vi "Report_backup.vi"(6 "Func ctl":enum16{"Backup Report", "Recover Report"}(ring), 8 "error in":errorcluster, 11 "DUT?":string="DUT1") -> (0 "error out":errorcluster)   [LabVIEW 2012]
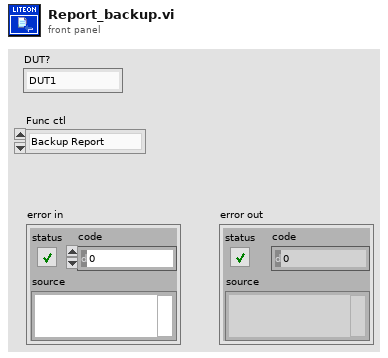
[diagram p1: front panel]
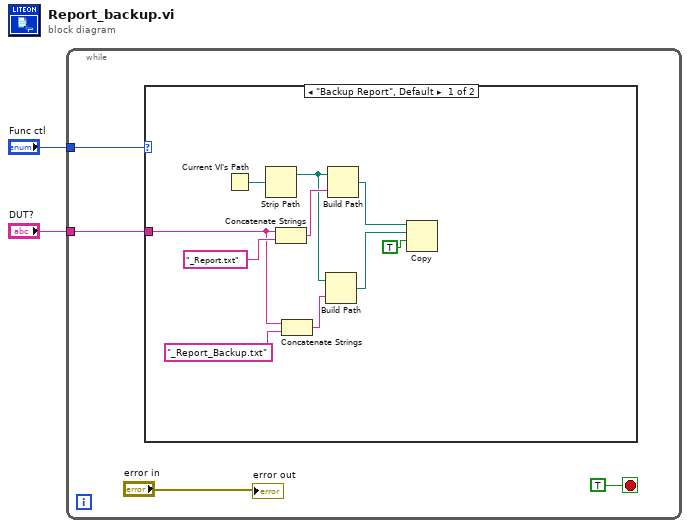
[diagram p0: block diagram]
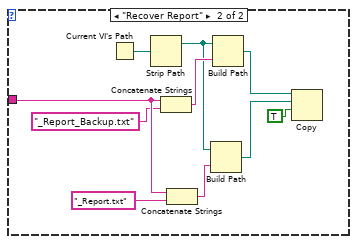
[diagram p2: hidden frame]
diagram:
  n1 = while {
    tunnel: "Func ctl" -> [w5]
    tunnel: "DUT?" -> [w4]
    stop <- TRUE stop-if-true
    n2 = case shown="\"Backup Report\", Default" w5 {
      tunnel: w4 -> [w7 w19]
      frame "Backup Report", Default {
        n3 = Current VI's Path() -> (path=w16:path)
        n4 = Strip Path(path=w16) -> (stripped path=w12:path)  [unwired: 1 out]
        n5 = Concatenate Strings(w7, "_Report.txt" ("string")) -> (w13:string)
        n6 = Concatenate Strings(w7, "_Report_Backup.txt" ("string")) -> (w11:string)
        n7 = Build Path(base path=w12, name or relative path=w11) -> (appended path=w9:path)
        n8 = Build Path(base path=w12, name or relative path=w13) -> (appended path=w10:path)
        n9 = Copy(9:TRUE ("overwrite (F)"), 10:w9, 11:w10) -> ()  [unwired: 2 in, 3 out]
      }
      frame "Recover Report" {
        n10 = Current VI's Path() -> (path=w26:path)
        n11 = Strip Path(path=w26) -> (stripped path=w24:path)  [unwired: 1 out]
        n12 = Concatenate Strings(w19, "_Report_Backup.txt" ("string")) -> (w25:string)
        n13 = Concatenate Strings(w19, "_Report.txt" ("string")) -> (w23:string)
        n14 = Build Path(base path=w24, name or relative path=w23) -> (appended path=w21:path)
        n15 = Build Path(base path=w24, name or relative path=w25) -> (appended path=w22:path)
        n16 = Copy(9:TRUE ("overwrite (F)"), 10:w21, 11:w22) -> ()  [unwired: 2 in, 3 out]
      }
    }
    "error out" <- "error in"
  }
